vi "hack_scene_reference_copy.vi"(10 "Object   Orig In":refnum<vi>) -> (1 "Object Copy Out":refnum<vi>, 2 "Object Orig Out":refnum<vi>)   [LabVIEW 2020, in "3DPC_SurfacePlot.xctl"]
uses:
  <vilib>/Native 3D Graph/xcontrol/3DPC_SurfacePlot.xctl
  <vilib>/picture/3D Picture Control/Object/Create Object (name).vi
  <vilib>/picture/3D Picture Control/NI_3D Picture Control.lvlib
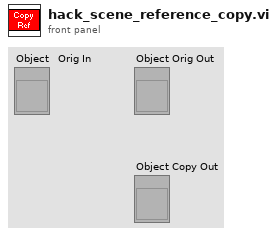
[diagram p1: front panel]
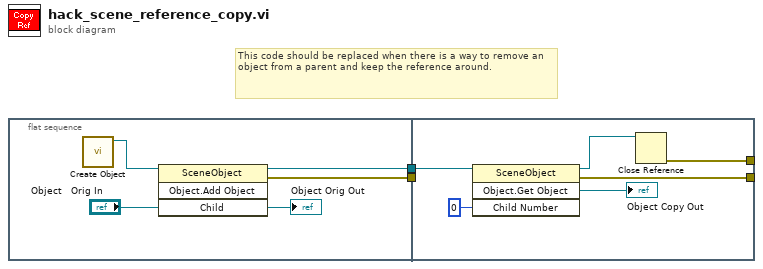
[diagram p0: block diagram]
diagram:
  # "This code should be replaced when there is a way to remove an object from a parent and keep the reference around."
  n1 = flat-sequence {
    tunnel: [w5] -> w2
    tunnel: [w3] -> w1
    tunnel: w2 -> [w13]
    tunnel: w1 -> [_]
    tunnel: [w9] -> _
    tunnel: [w8] -> _
    frame #0 {
      n2 = call-poly <vilib>:"Create Object.vi"() -> ("Scene:New Object"=w7:refnum<vi>)  [unwired: 10 in, 1 out]
      n3 = invoke class="SceneObject" method="Object.Add Object"(reference=w7, "Child"="Object   Orig In") -> (reference out=w5:refnum<vi>, error out=w3:errorcluster, "Child"=→"Object Orig Out":refnum<vi>)  [unwired: 2 in, 1 out]
    }
    frame #1 {
      n4 = invoke class="SceneObject" method="Object.Get Object"(reference=w13, "Child Number"=0 ("index")) -> (reference out=w10:refnum<vi>, error out=w9:errorcluster, "Get Child"=→"Object Copy Out":refnum<vi>)  [unwired: 2 in, 1 out]
      n5 = Close Reference(reference=w10) -> (error out=w8:errorcluster)  [unwired: 1 in]
    }
  }
